vi "Graphs.vi"() -> ()   [LabVIEW 2018]
uses:
  <vilib>/Instr/_visa.llb/VISA Configure Serial Port (Instr).vi
panel:
  in  "stop":bool
  out "Temp":dynamicdata(graph)
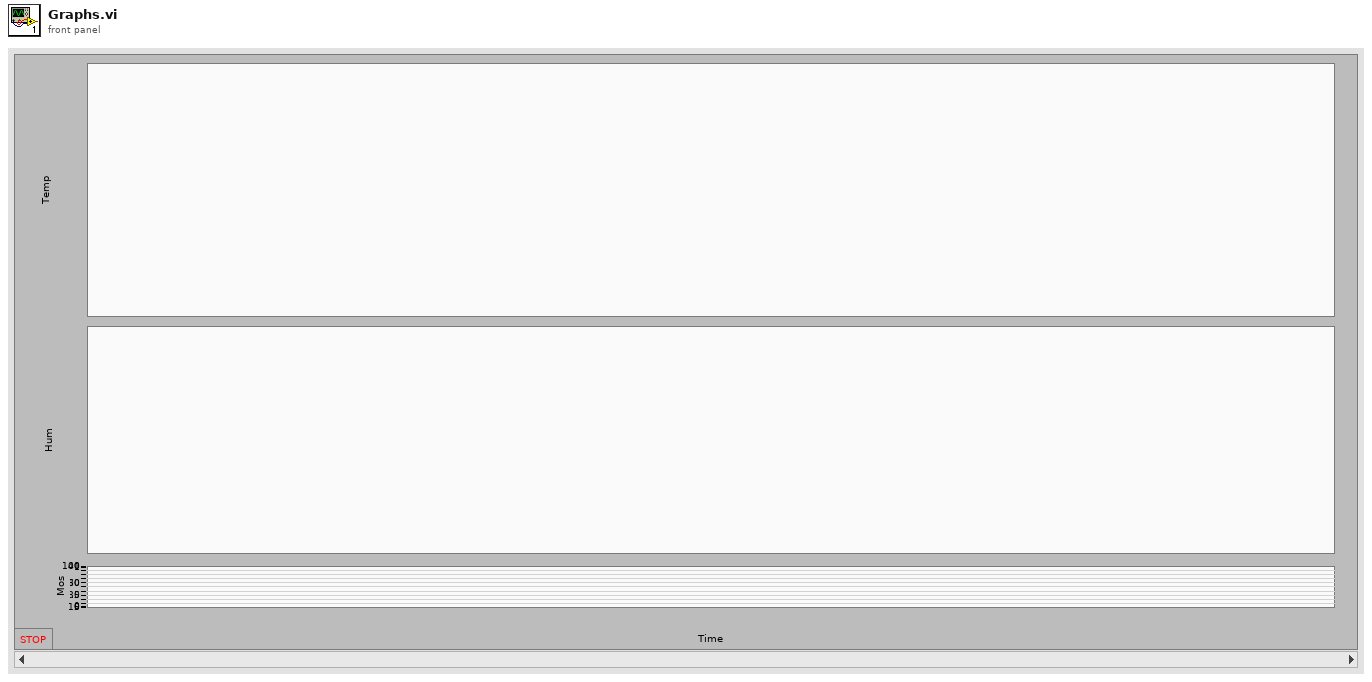
[diagram p1: front panel]
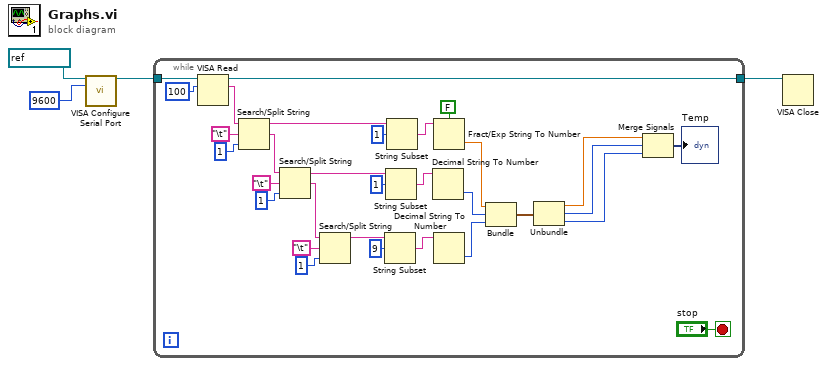
[diagram p0: block diagram]
diagram:
  n1 = call-poly "VISA Configure Serial Port"("VISA resource name"=refnum<visa-resource-name> "COM5", "baud rate (9600)"=u32 9600) -> ("VISA resource name out"=w2:refnum<visa-resource-name>)  [unwired: 12 in, 1 out]
  n2 = while {
    tunnel: w2 -> [w34]
    tunnel: [w35] -> w3
    stop <- "stop" stop-if-true
    n3 = VISA Read(VISA resource name=w34, byte count=u32 100) -> (VISA resource name out=w35:refnum<visa-resource-name>, read buffer=w22:string)  [unwired: 1 in, 2 out]
    n4 = Search/Split String(string=w22, search string/char (-)="\t", offset (0)=1) -> (substring before match=w13:string, match + rest of string=w17:string)  [unwired: 1 out]
    n5 = Search/Split String(string=w17, search string/char (-)="\t", offset (0)=1) -> (substring before match=w7:string, match + rest of string=w14:string)  [unwired: 1 out]
    n6 = Search/Split String(string=w14, search string/char (-)="\t", offset (0)=1) -> (substring before match=w8:string)  [unwired: 2 out]
    n7 = String Subset(string=w8, offset (0)=9) -> (substring=w5:string)  [unwired: 1 in]
    n8 = String Subset(string=w7, offset (0)=1) -> (substring=w6:string)  [unwired: 1 in]
    n9 = String Subset(string=w13, offset (0)=1) -> (substring=w12:string)  [unwired: 1 in]
    n10 = Decimal String To Number(string=w6) -> (number=w29:i32)  [unwired: 2 in, 1 out]
    n11 = Fract/Exp String To Number(use system decimal point (T)=FALSE, string=w12) -> (number=w30:dbl)  [unwired: 2 in, 1 out]
    n12 = Decimal String To Number(string=w5) -> (number=w28:i32)  [unwired: 2 in, 1 out]
    n13 = Bundle(w30, w29, w28) -> (w26:cluster{dbl, i32, i32})  [unwired: 1 in]
    n14 = Unbundle(w26) -> (w27:dbl, w25:i32, w24:i32)
    n15 = Merge Signals(w27, w25, w24) -> (→"Temp":dynamicdata)
  }
  n16 = VISA Close(VISA resource name=w3) -> ()  [unwired: 1 in, 1 out]
